vi "SP - click.vi"(8 "error in (no error)":errorcluster, 11 "JSON string":string) -> (0 "error out":errorcluster, 3 "value":string)   [LabVIEW 2020, in "ui-testing.lvlib"]
doc: "copyright: Thomas Zilliox©"
uses:
  ui-testing.lvlib
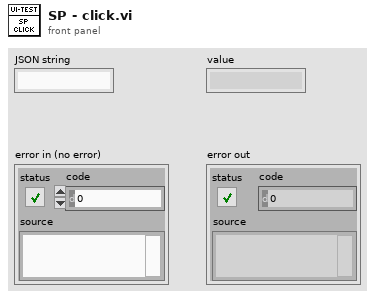
[diagram p1: front panel]
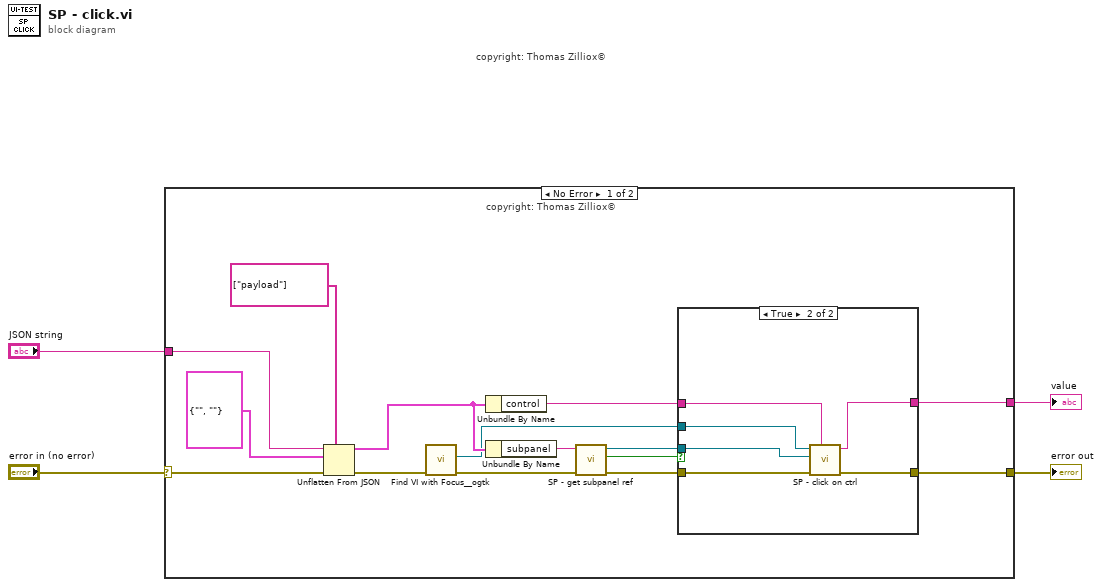
[diagram p0: block diagram]
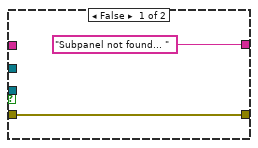
[diagram p2: hidden frame]
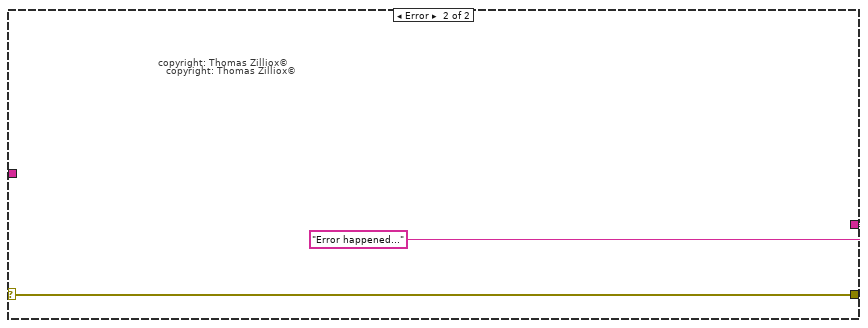
[diagram p3: hidden frame]
diagram:
  # "copyright: Thomas Zilliox©"
  n1 = case shown="No Error" "error in (no error)" {
    selector: "error in (no error)" -> [w15 w29]
    tunnel: "JSON string" -> [w17 _]
    tunnel: [w16 w29] -> w3
    tunnel: [w12 "Error happened..."] -> w1
    frame No Error {
      # "copyright: Thomas Zilliox©"
      n2 = Unflatten From JSON(path=string[] ["payload"], JSON string=w17, type and defaults=cluster{"subpanel":string, "control":string} {"subpanel"="", "control"=""}, error in (no error)=w15) -> (value=w13:cluster{"subpanel":string, "control":string}, error out=w18:errorcluster)  [unwired: 3 in]
      n3 = call <userlib>:"Find VI with Focus__ogtk.vi"("error in"=w18) -> ("error out"=w7:errorcluster, "VI with Focus"=w6:refnum<vi>)  [unwired: 6 in, 3 out]
      n4 = Unbundle By Name(w13) -> ("control"=w9:string)
      n5 = Unbundle By Name(w13) -> ("subpanel"=w11:string)
      n6 = call "SP - get subpanel ref.vi"("error in (no error)"=w7, "subpanel"=w11) -> ("error out"=w10:errorcluster, "subpanel found ?"=w5:bool, "subpanel VI ref"=w8:refnum<vi>)  [unwired: 6 in, 1 out]
      n7 = case shown="True" w5 {
        tunnel: [w21 w26] -> w16
        tunnel: w8 -> [_ w24]
        tunnel: w10 -> [w21 w22]
        tunnel: w9 -> [_ w23]
        tunnel: ["Subpanel not found... " ("result string") w27] -> w12
        tunnel: w6 -> [_ w25]
        frame False {
        }
        frame True {
          n8 = call "SP - click on ctrl.vi"("Control Label"=w23, "error in (no error)"=w22, "subVI"=w24, "VI with Focus"=w25) -> ("error out"=w26:errorcluster, "return value"=w27:string)  [unwired: 6 in]
        }
      }
    }
    frame Error {
      # "copyright: Thomas Zilliox©"
      # "copyright: Thomas Zilliox©"
    }
  }
  "error out" <- w3
  "value" <- w1
